vi "RawToScaled.vi"(8 "error in (no error)":errorcluster, 10 "RAW":dbl, 11 "Scale in":refnum<class "Scale.lvclass">) -> (0 "error out":errorcluster, 2 "Scaled":dbl, 3 "Scale out":refnum<class "Scale.lvclass">)   [LabVIEW 2019, in "Scale.lvclass"]
uses:
  Scale.lvclass
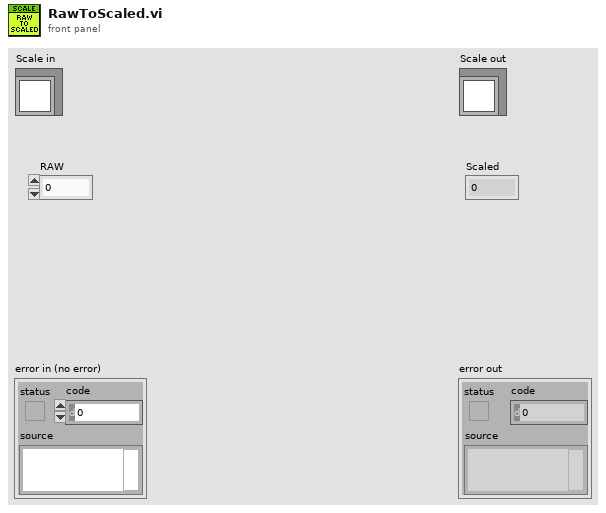
[diagram p1: front panel]
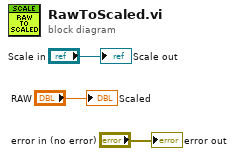
[diagram p0: block diagram]
diagram:
  "error out" <- "error in (no error)"
  "Scale out" <- "Scale in"
  "Scaled" <- "RAW"
